vi "SynchronousPump_TwoCommands.vi"(6 "Command 2":string, 7 "Command 1":string, 8 "error in (no error)":errorcluster, 10 "Pump #":dbl, 11 "VISA Refnum in":refnum<visa-resource-name>) -> (0 "error out":errorcluster, 1 "Read (Response) 2":string, 2 "Read (Response)":string, 3 "VISA resource name out":refnum<visa-resource-name>, 4 "EXIT PROGRAM? (F)":bool)   [LabVIEW 2013]
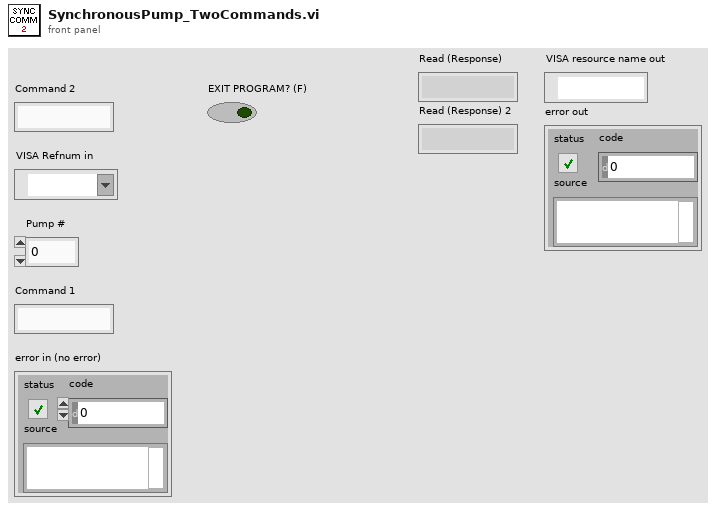
[diagram p1: front panel]
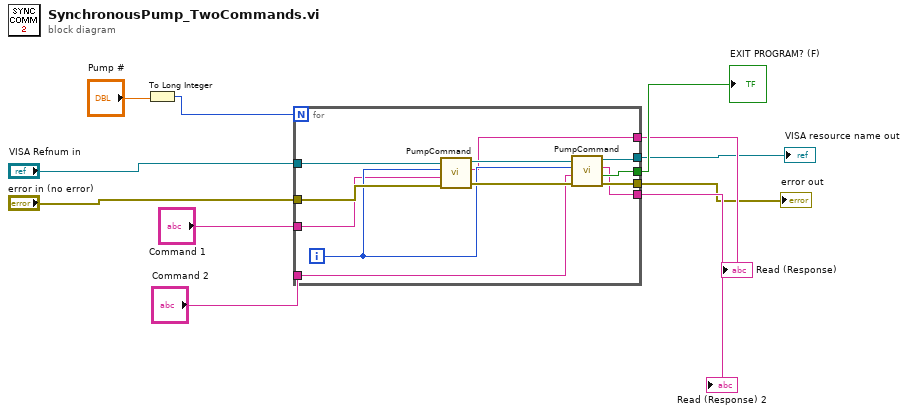
[diagram p0: block diagram]
diagram:
  n1 = To Long Integer(number="Pump #") -> (32bit integer=w2:i32)
  n2 = for {
    N: w2 -> [_]
    tunnel: "VISA Refnum in" -> [w21]
    tunnel: "error in (no error)" -> [w20]
    tunnel: [w18] -> w9
    tunnel: "Command 1" -> [w17]
    tunnel: [w16] -> w4
    tunnel: [w15] -> w3
    tunnel: "Command 2" -> [w14]
    tunnel: [w13] -> w6
    tunnel: [w12] -> w5
    i -> [w19]
    n3 = call "PumpCommand.vi"("error in (no error)"=w20, "Command:"=w17, "Pump Address"=w19, "VISA Refnum in"=w21) -> ("error out"=w23:errorcluster, "Read (Response)"=w13:string, "VISA resource name out"=w22:refnum<visa-resource-name>)  [unwired: 3 in, 1 out]
    n4 = call "PumpCommand.vi"("error in (no error)"=w23, "Command:"=w14, "Pump Address"=w19, "VISA Refnum in"=w22) -> ("error out"=w15:errorcluster, "EXIT PROGRAM? (F)"=w18:bool, "Read (Response)"=w12:string, "VISA resource name out"=w16:refnum<visa-resource-name>)  [unwired: 3 in]
  }
  "EXIT PROGRAM? (F)" <- w9
  "Read (Response)" <- w6
  "Read (Response) 2" <- w5
  "VISA resource name out" <- w4
  "error out" <- w3
